vi "ZAlign_AlignLocalControls.vi"(8 "error in (no error)":errorcluster, 9 "Max right location":u32, 10 "CtrlRefs":refnum<vi>[](array[refnum]) caption="Array", 11 "Panel in":refnum<vi>) -> (0 "error out":errorcluster, 1 "Bottom":u32, 2 "Left":u32, 3 "Max Right":u32)   [LabVIEW 2014, in "ZAlign.lvlib"]
doc: "ZAlign.lvlib:ZAlign_AlignLocalControls.vi\n----------------------------------------------\nAlign Local Controls\n\nInputs:\n---------------------\n- error in (no error) : Cluster; \n- Max right location : U32; \n- Array : 1DArrayOfRefnum; \n- Panel in : Refnum; \n\nOutputs:\n---------------------\n- error out : Cluster; \n- Bottom : U32; \n- Left : U32; \n- Max Right : U32; \n\n----------------------------------------------\n16/03/2015\nZühlke Engineering AG\nCH-8952 Schlieren\nwww.zuehlke.com"
uses:
  ZAlign.lvlib
panel:
  # "Connector Pane"
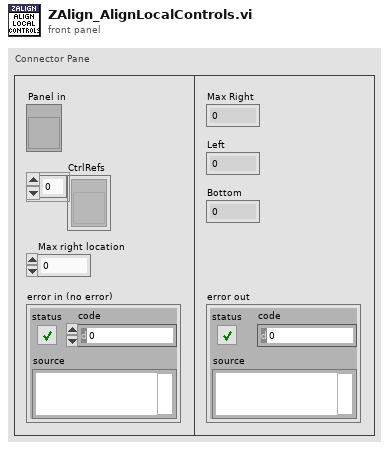
[diagram p1: front panel]
types:
  T1 = typedef "LVPositionTypeDef.ctl" = cluster{"Left":i32, "Top":i32}
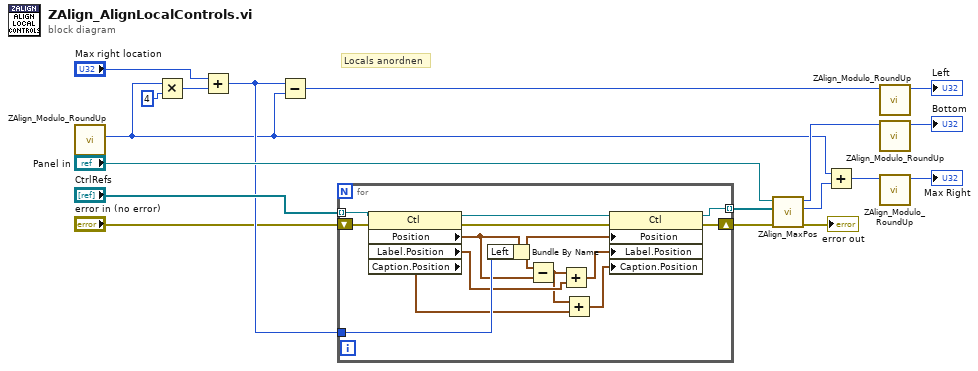
[diagram p0: block diagram]
diagram:
  # "Locals anordnen"
  n1 = call "ZAlign_Modulo_RoundUp.vi"() -> ("Grid_Size"=w3:i32)  [unwired: 10 in, 1 out]
  n2 = Multiply(x=w3, y=i16 4) -> (x*y=w18:i32)
  n3 = Add(x="Max right location", y=w18) -> (x+y=w10:u32)
  n4 = Subtract(x=w10, y=w3) -> (x-y=w8:u32)
  n5 = for {
    tunnel: "CtrlRefs" -> [w32] mode=indexing
    tunnel: [w29] -> w13 mode=indexing
    tunnel: w10 -> [w26]
    shift-right: [w27] -> w14
    shift-left: "error in (no error)" -> [w31]
    n6 = property class="Ctl"(reference=w32, error in=w31) -> (reference out=w30:refnum<vi>, error out=w28:errorcluster, "Position"=w24:T1, "Label.Position"=w23:T1, "Caption.Position"=w20:T1)
    n7 = Bundle By Name(cluster=w24, "Left"=w26) -> (w25:T1)
    n8 = Subtract(x=w25, y=w24) -> (x-y=w21:T1)
    n9 = Add(x=w21, y=w23) -> (x+y=w22:T1)
    n10 = Add(x=w21, y=w20) -> (x+y=w19:T1)
    n11 = property class="Ctl"(reference=w30, error in=w28, "Position"=w25, "Label.Position"=w22, "Caption.Position"=w19) -> (reference out=w29:refnum<vi>, error out=w27:errorcluster)
  }
  n12 = call "ZAlign_MaxPos.vi"("error in (no error)"=w14, "Objects"=w13, "Panel"="Panel in") -> ("error out"=→"error out":errorcluster, "Max right location"=w2:u32, "Height"=w4:u32)  [unwired: 6 in]
  n13 = Add(x=w3, y=w2) -> (x+y=w1:u32)
  n14 = call "ZAlign_Modulo_RoundUp.vi"("Value in"=w8) -> ("Value out"=→"Left":i32)  [unwired: 9 in, 1 out]
  n15 = call "ZAlign_Modulo_RoundUp.vi"("Value in"=w4) -> ("Value out"=→"Bottom":i32)  [unwired: 9 in, 1 out]
  n16 = call "ZAlign_Modulo_RoundUp.vi"("Value in"=w1) -> ("Value out"=→"Max Right":i32)  [unwired: 9 in, 1 out]
